vi "CloseConnectionToServer.vi"(3 "TCP Network Connection Refnum":refnum<k5>) -> ()   [LabVIEW 2012]
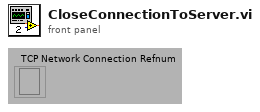
[diagram p1: front panel]
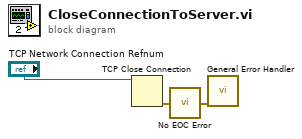
[diagram p0: block diagram]
diagram:
  n1 = TCP Close Connection(connection ID="TCP Network Connection Refnum") -> (error out=w3:errorcluster)  [unwired: 1 in, 2 out]
  n2 = call "No EOC Error.vi"("error in"=w3) -> ("error out"=w2:errorcluster)  [unwired: 4 out]
  n3 = call <vilib>:"General Error Handler.vi"("error in (no error)"=w2) -> ()  [unwired: 1 in, 14 out]
